vi "CPP_TubingCorrectionFromCrossSpectra.vi"() -> (5 "Plug in titles":string[](array[string]), 7 "Plug in values":string[](array[string]))   [LabVIEW 2012]
uses:
  Globals/Meas_global.vi
  <vilib>/Analysis/baseanly.llb/Mean (DBL).vi
  Plug in sub vis/CPP_TubingCompensation/AudioGlobal.vi
  <vilib>/Analysis/NI_AALPro.lvlib
  <vilib>/Analysis/NI_AALBase.lvlib
panel:
  in  "ArbitraryTestGraphShift":dbl(slide)=1.0 scale=1e-06..1000000.0
  out "CutoffFrequencyUsed":dbl=15.0
  out "MaxBoostUsed":dbl=15.0
  in  "CutoffFrequency":dbl=200.0
  in  "MaxBoost":dbl=15.0
  out "TimeSeries":cluster{dbl, dbl, dbl[]}[](graph)
  in  "Ref":i32(ring) items=["RV (1.0Naked)", "RV (5.0Naked)", "RV (0.75Naked)"]
  in  "Test":i32(ring) items=["RV (1.0Naked)", "RV (5.0Naked)", "RV (0.75Naked)"]
  out "Spectra":cluster{dbl, dbl, dbl[][]}(graph)
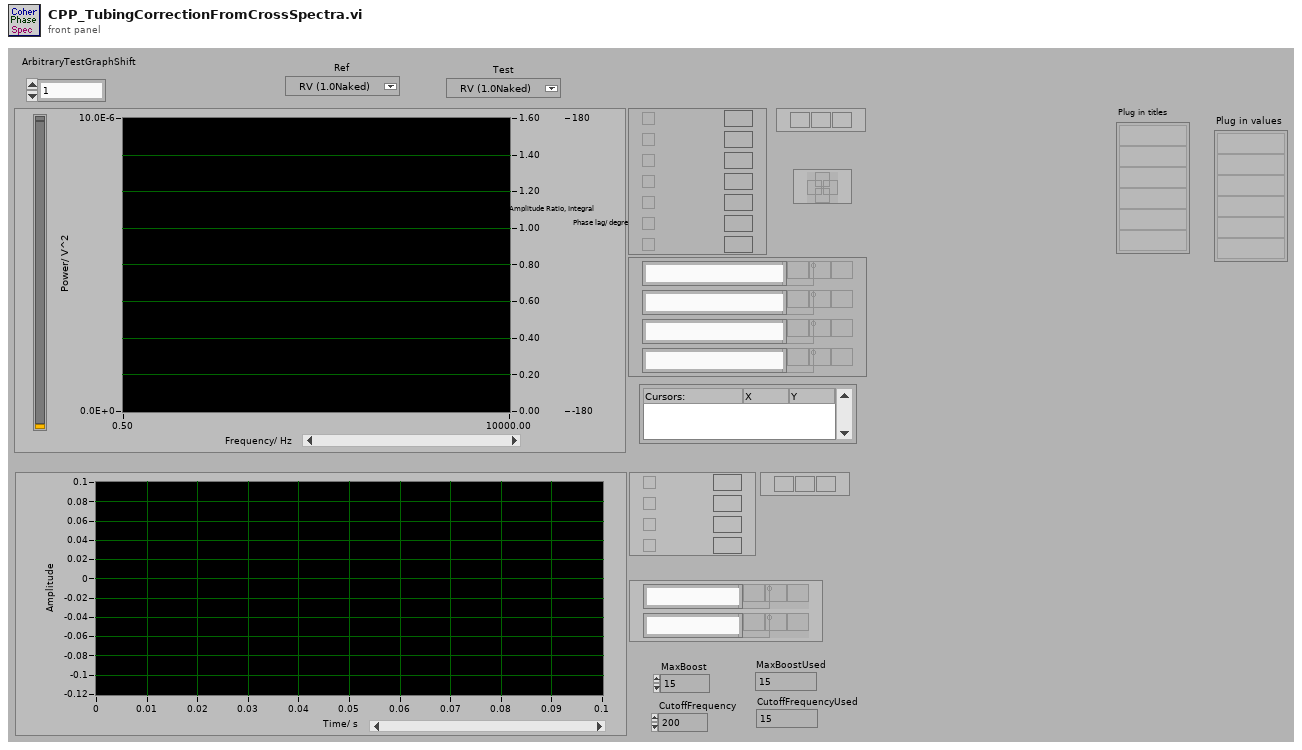
[diagram p1: front panel]
types:
  T1 = typedef "Analysis_info_cluster.ctl" = cluster{"Colour":u32, "Inst type":T2, "Inst name":string, "Symbol":string, "Code name":string, "Extra Info":string, "Inst Array":T3, "Extra Titles":string[], "Extra Values":string[], "U":dbl, "u^2":dbl, "u^3":dbl, "u^4":dbl, "Skew_u":dbl, "Kurt_u":dbl, "Sd Error in Mean":dbl, "% u'/U":dbl, "X":dbl, "Y":dbl, "Z":dbl, "Timescale integral to 25%":dbl, "Sd Error in Variance":dbl, "Calib File":path, "Calib Constants":dbl[], "Output Position":bool, "Full Stats":bool, "Av Sampling Rate":dbl, "Av No of Samples":dbl, "Total Meas Time (s)":dbl, "ADAM Ch Name":string}
  T2 = typedef "Inst_type.ctl" = enum16{"Propeller anemometer", "Raw voltage", "Pressure Transducer", "Pitot-static tube", "Preston tube", "Hot wire", "Cross wire 1", "Cross wire 2", "Generic Linear", "Generic Polynomial", "Generic BackPoly", "Fast FID", "Thermocouple", "Cold wire", "Pulsed Wire", "LDA Vel", "LDA Tran time", "LDA Arr time"}
  T3 = typedef "Instrument_Array.ctl" = enum16{"PWA", "LDA", "Analogue"}
  T4 = typedef "Time_Trace_Cluster.ctl" = cluster{"Weighting":dbl[], "Time (s)":dbl[], "Voltage":dbl[], "Eng Values":dbl[]}
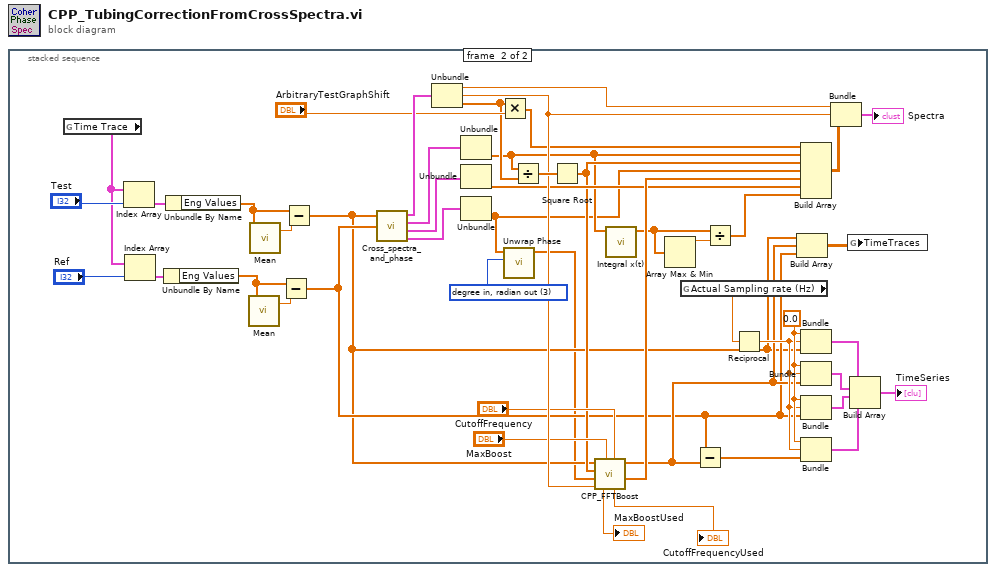
[diagram p0: block diagram]
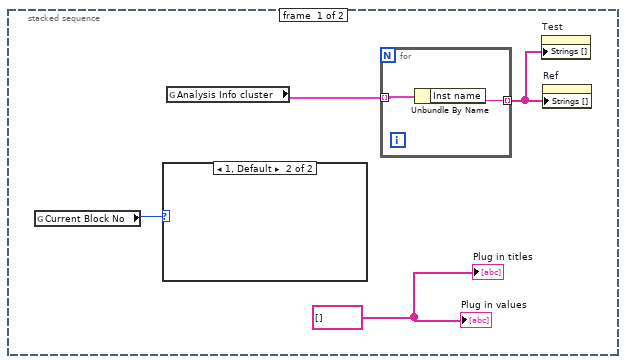
[diagram p2: hidden frame]
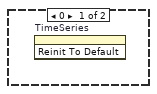
[diagram p3: hidden frame]
diagram:
  n1 = stacked-sequence {
    frame #0 {
      w2 = string[] [] ("Add in values")
      n2 = global read "Meas_global.vi" "Current Block No"() -> (w1:i32)
      n3 = case shown="1, Default" w1 {
        frame 0 {
          n4 = invoke on="TimeSeries" class="WFGraph (strict)" method="Reinit To Default"() -> ()  [unwired: 3 in, 3 out]
        }
        frame 1, Default {
        }
      }
      n5 = global read "Meas_global.vi" "Analysis Info cluster"() -> (w4:T1[])
      n6 = for {
        tunnel: w4 -> [w6] mode=indexing
        tunnel: [w5] -> w3 mode=indexing
        n7 = Unbundle By Name(w6) -> ("Inst name"=w5:string)
      }
      n8 = property on="Test" class="Ring (strict)"("Strings []"=w3) -> ()  [unwired: 2 in, 2 out]
      n9 = property on="Ref" class="Ring (strict)"("Strings []"=w3) -> ()  [unwired: 2 in, 2 out]
      "Plug in titles" <- w2
      "Plug in values" <- w2
    }
    frame #1 {
      w28 = 0.0
      w46 = 3 items=["radian in, radian out", "radian in, degree out", "degree in, degree out", "degree in, radian out"] ("phase unit")
      n10 = global read "Meas_global.vi" "Time Trace"() -> (w32:T4[])
      n11 = Index Array(array=w32, index="Test") -> (element=w42:T4)
      n12 = Index Array(array=w32, index="Ref") -> (element=w30:T4)
      n13 = Unbundle By Name(w30) -> ("Eng Values"=w29:dbl[])
      n14 = Unbundle By Name(w42) -> ("Eng Values"=w31:dbl[])
      n15 = call-poly <vilib>:"Mean.vi"("X"=w29) -> ("mean"=w43:dbl)  [unwired: 1 out]
      n16 = call-poly <vilib>:"Mean.vi"("X"=w31) -> ("mean"=w44:dbl)  [unwired: 1 out]
      n17 = Subtract(x=w29, y=w43) -> (x-y=w17:dbl[])
      n18 = Subtract(x=w31, y=w44) -> (x-y=w16:dbl[])
      n19 = call "Cross_spectra_and_phase.vi"("U1"=w16, "U2"=w17) -> ("U1 spectra"=w52:cluster{dbl, dbl, dbl[]}, "U2 spectra"=w51:cluster{dbl, dbl, dbl[]}, "U1 U2 coherence"=w34:cluster{dbl, dbl, "Coherence array":dbl[]}, "U1 U2 phase"=w47:cluster{dbl, dbl, "Phase array":dbl[]})  [unwired: 3 out]
      n20 = Unbundle(w52) -> (w49:dbl, w41:dbl, w14:dbl[])
      n21 = Unbundle(w51) -> (w12:dbl[])  [unwired: 2 out]
      n22 = Unbundle(w34) -> ("Coherence array"=w33:dbl[])  [unwired: 2 out]
      n23 = Unbundle(w47) -> ("Phase array"=w11:dbl[])  [unwired: 2 out]
      n24 = Multiply(x=w14, y="ArbitraryTestGraphShift") -> (x*y=w13:dbl[])
      n25 = call <vilib>:"Unwrap Phase.vi"("phase unit"=w46, "Phase"=w11) -> ("Unwrapped Phase"=w10:dbl[])  [unwired: 8 in, 1 out]
      n26 = Divide(x=w12, y=w14) -> (x/y=w45:dbl[])
      n27 = Square Root(x=w45) -> (sqrt(x)=w21:dbl[])
      n28 = call "CPP_FFTBoost.vi"("CutoffFrequency"="CutoffFrequency", "MaxBoost"="MaxBoost", "dF"=w41, "UnwrappedPhaseLag"=w10, "AmplitudeBoost"=w21, "Muffleddata"=w16) -> ("BandLimitedBoost"=w36:dbl[], "boostedData"=w18:dbl[], "CutoffFrequencyUsed"=→"CutoffFrequencyUsed":dbl, "MaxBoostUsed"=→"MaxBoostUsed":dbl)  [unwired: 2 in]
      n29 = call <vilib>:"Integral x(t).vi"("X"=w12) -> ("Integral X"=w9:dbl[])  [unwired: 9 in, 1 out]
      n30 = Array Max & Min(array=w9) -> (max value=w7:dbl)  [unwired: 3 out]
      n31 = global read "Meas_global.vi" "Actual Sampling rate (Hz)"() -> (w35:dbl)
      n32 = Subtract(x=w17, y=w18) -> (x-y=w19:dbl[])
      n33 = Divide(x=w9, y=w7) -> (x/y=w8:dbl[])
      n34 = Reciprocal(x=w35) -> (1/x=w22:dbl)
      n35 = Build Array(w16, w18, w17) -> (w20:dbl[][])
      n36 = Build Array(w13, w12, w21, w11, w36, w33, w8) -> (w50:dbl[][])
      n37 = Bundle(w28, w22, w16) -> (w27:cluster{dbl, dbl, dbl[]})  [unwired: 1 in]
      n38 = Bundle(w28, w22, "boostedData"=w18) -> (w24:cluster{dbl, dbl, "boostedData":dbl[]})  [unwired: 1 in]
      n39 = Bundle(w28, w22, w17) -> (w25:cluster{dbl, dbl, dbl[]})  [unwired: 1 in]
      n40 = Bundle(w28, w22, w19) -> (w26:cluster{dbl, dbl, dbl[]})  [unwired: 1 in]
      n41 = Bundle(w49, w41, w50) -> (→"Spectra":cluster{dbl, dbl, dbl[][]})  [unwired: 1 in]
      n42 = global write "AudioGlobal.vi" "TimeTraces"(w20) -> ()
      n43 = Build Array(w27, w24, w25, w26) -> (→"TimeSeries":cluster{dbl, dbl, "boostedData":dbl[]}[])
    }
  }
